vi "Interactive Demo.vi"() -> ()   [LabVIEW 2013, in "dotNETChart XControl.xctl"]
uses:
  dotNETChart XControl.xctl
  typedefs/ChartType.ctl
  typedefs/3DSettings.ctl
  <vilib>/express/express shared/transition.llb/Dynamic To Waveform Array.vi
  <vilib>/express/express signal manip/GetorSetDDTAttributes/Set DDT Attributes/SetT0.vi
  <vilib>/express/express shared/transition.llb/Waveform Array To Dynamic.vi
  <vilib>/express/express signal manip/GetorSetDDTAttributes/Set DDT Attributes/Set DDT Properties.xnode
panel:
  in  "Chart Type 2":i32(ring)=4 caption="Chart Type"
  in  "Series 1 Data Colour":u32(colorbox)=6836 caption="Series Data Colour"
  in  "series name":string="First Series Title" caption="xaxislabel"
  in  "Chart Palette":u16(ring)
  in  "Chart Type":i32(ring)=4
  in  "Chart Wall Gradient Colour":u32(colorbox)=12116479
  in  "Gradient Style":i32(ring)=4
  in  "Chart Wall Border Colour":u32(colorbox)=16777238
  in  "Chart Wall Colour":u32(colorbox)
  in  "chart_wall_trans":u8(slide)=31 caption="Chart Wall Opacity" scale=0.0..255.0
  in  "Legend Style":u16(ring) items=["Column", "Row", "Table"]
  in  "Mouse Zoom":u16(ring)=1 items=["off", "on (2D mode only)"]
  in  "Series 2 Data Colour":u32(colorbox)=12116479 caption="Series Data Colour"
  in  "Skin Style":i32(ring)=1 items=["None", "Emboss", "Raised", "Sunken", "FrameThin1", "FrameThin2", "FrameThin3", "FrameThin4", "FrameThin5", "FrameThin6", "FrameTitle1", "FrameTitle2", "FrameTitle3", "FrameTitle4", "FrameTitle5", "FrameTitle6", "FrameTitle7", "FrameTitle8"]
  in  "yaxislabel":string="Y axis label" caption="xaxislabel"
  in  "xaxislabel":string="X axis label"
  in  "3dmode":bool=TRUE caption="3D Mode"
  in  "Rotation":i32=25
  in  "Wall Width":i32=2
  in  "Perspective":i32=4
  in  "LightStyle":i32(ring)=2 items=["None", "Simplistic", "Realistic"]
  in  "Inclination":i32=21
  in  "Random":bool
  out "dotNETChart XControl":dynamicdata(xcontrol)=[{"t0"=timestamp(3359225754.779551 s since 1904-01-01), "dt"=0.001, "Y"=[-0.21293878372691832, 0.10480719171607178, 0.5198645121842703, 0.4960927860135643, 0.8486500407057044, -0.19156178243419908, -0.3213988951228298, -1.0007275322775073, -1.3720240757016509, -0.2660093892305525, -0.23724681626115568, 0.796814395938406, 0.9778645666014882, 0.7870343306028441, 0.7585739928106939, 0.26409213430431566, -0.8946529385336436, -1.169162891258134, -1.1556662975978256, -0.3690681531689127], "attributes"=variant("NI_ChannelName"=variant(string "First Series Title"), "NI_ExpIsRelativeTime"=variant(bool FALSE), "NI_ExpStartTimeStamp"=variant(timestamp timestamp(3359225754.779551 s since 1904-01-01)), "NI_ExpTimeStamp"=variant(timestamp timestamp(3359225754.779551 s since 1904-01-01)), "NI_ExpXDimension"=variant(string "t"))}, {"t0"=timestamp(3359225754.779551 s since 1904-01-01), "dt"=0.001, "Y"=[-0.22651223041771185, 0.4171889778375242, 0.6017245565566697, 0.9588615672567297, 0.748101089941119, -0.27993796654087566, -0.8863552944000307, -1.0635191133061586, -0.9344284949437466, -0.1710474405944974, 0.3018910917348227, 0.5301156955284767, 1.4475242535659825, 1.1713473149513396, 0.25407740207025176, -0.025061984573477407, -0.48652113815437137, -0.7534989399164532, -1.2184058505207012, -0.10043002227520204], "attributes"=variant("NI_ChannelName"=variant(string "Sine with Uniform Noise"), "NI_ExpIsRelativeTime"=variant(bool FALSE), "NI_ExpStartTimeStamp"=variant(timestamp timestamp(3359225754.779551 s since 1904-01-01)), "NI_ExpTimeStamp"=variant(timestamp timestamp(3359225754.779551 s since 1904-01-01)), "NI_ExpXDimension"=variant(string "t"))}]
  # "Settings"
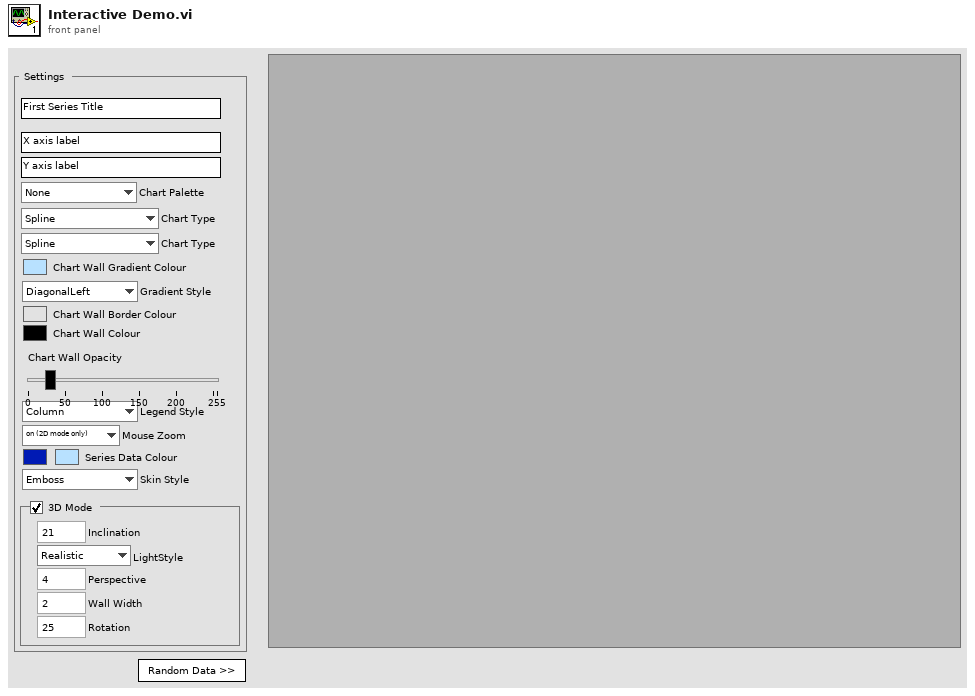
[diagram p1: front panel]
types:
  T1 = typedef "ChartType.ctl" = i32
  T2 = typedef "BackGradientStyle.ctl" = i32
  T3 = typedef "LegendStyle.ctl" = i32
  T4 = typedef "SkinStyle.ctl" = i32
  T5 = typedef "3DSettings.ctl" = cluster{"Inclination":i32, "LightStyle":i32, "Perspective":i32, "WallWidth":i32, "Rotation":i32}
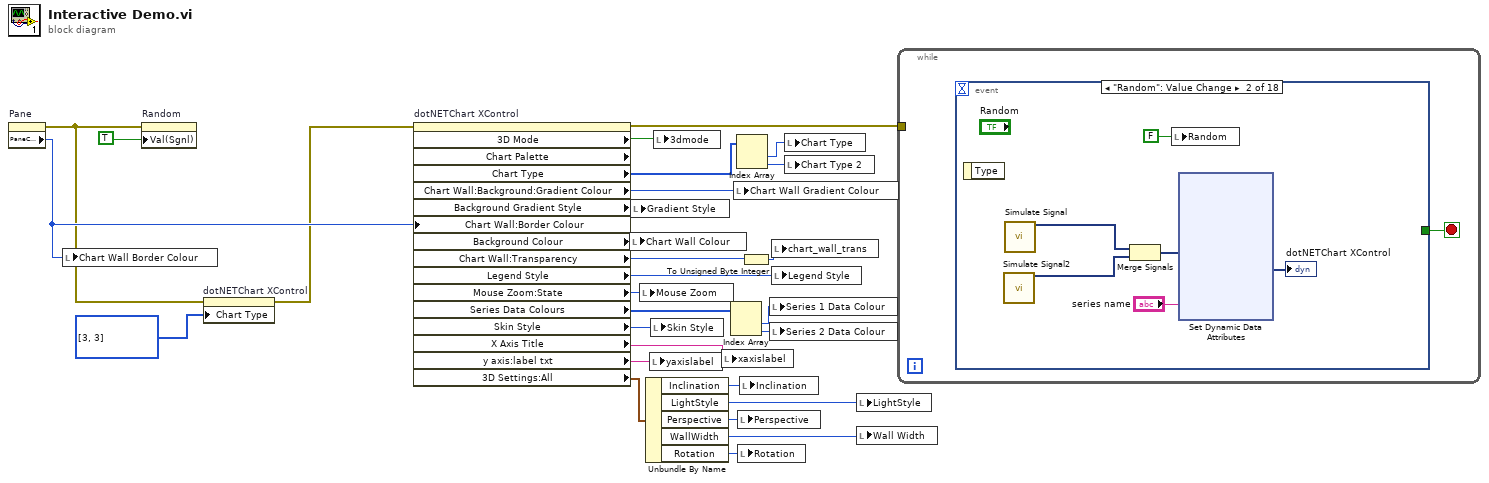
[diagram p0: block diagram]
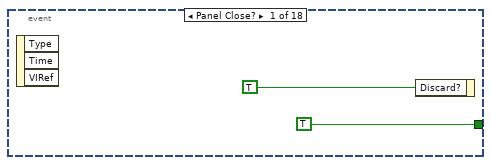
[diagram p2: hidden frame]
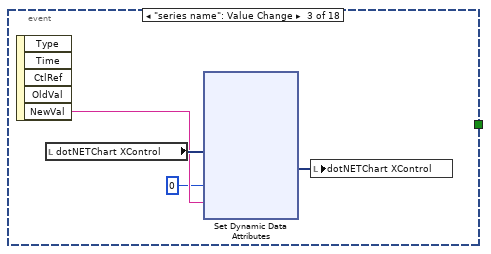
[diagram p3: hidden frame]
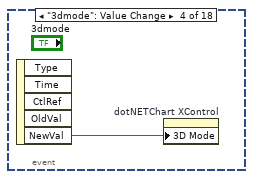
[diagram p4: hidden frame]
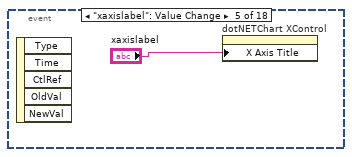
[diagram p5: hidden frame]
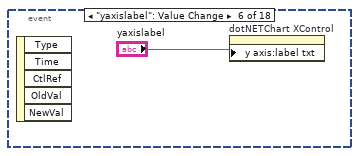
[diagram p6: hidden frame]
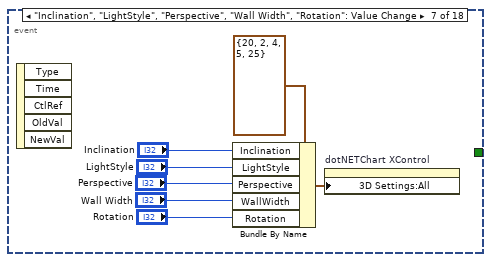
[diagram p7: hidden frame]
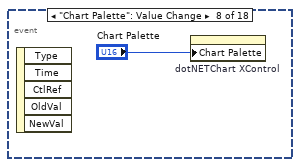
[diagram p8: hidden frame]
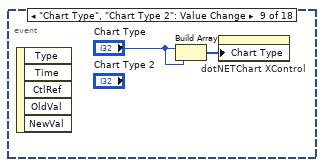
[diagram p9: hidden frame]
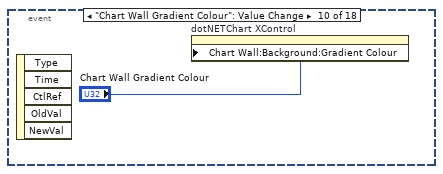
[diagram p10: hidden frame]
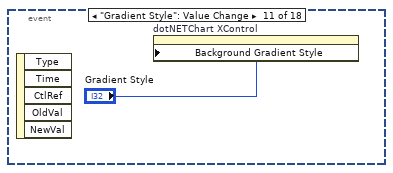
[diagram p11: hidden frame]
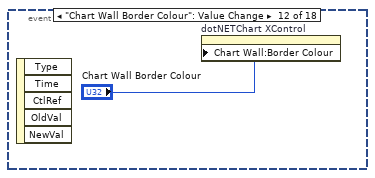
[diagram p12: hidden frame]
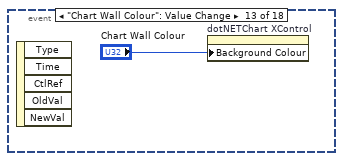
[diagram p13: hidden frame]
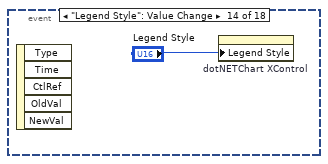
[diagram p14: hidden frame]
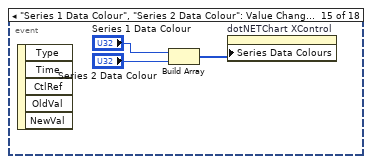
[diagram p15: hidden frame]
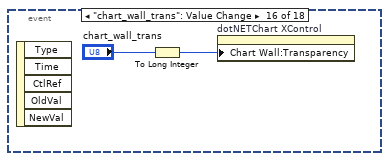
[diagram p16: hidden frame]
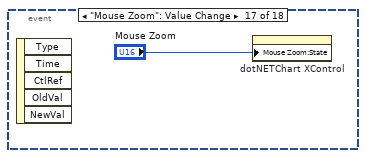
[diagram p17: hidden frame]
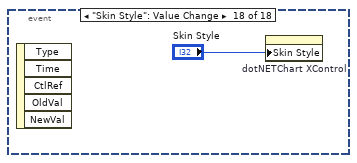
[diagram p18: hidden frame]
diagram:
  w2 = T1[] [3, 3] items=["Point", "FastPoint", "Bubble", "Line", "Spline", "StepLine", "FastLine", "Bar", "StackedBar", "StackedBar100", "Column", "StackedColumn", "StackedColumn100", "Area", "SplineArea", "StackedArea", "StackedArea100", "Pie", "Doughnut", "Stock", "Candlestick", "Range", "SplineRange", "RangeBar", "RangeColumn", "Radar", "Polar", "ErrorBar", "BoxPlot", "Renko", "ThreeLineBreak", "Kagi", "PointAndFigure", "Funnel", "Pyramid"] ("Chart Types")
  n1 = property on="Pane" class="Pane"() -> (error out=w3:errorcluster, "PaneColor"=w7:u32)  [unwired: 2 in, 1 out]
  n2 = local write "Chart Wall Border Colour"(w7) -> ()
  n3 = property on="Random" class="Bool (strict)"(error in=w3, "Val(Sgnl)"=TRUE ("Random")) -> ()  [unwired: 1 in, 2 out]
  n4 = property on="dotNETChart XControl" class="dotNETChart XControl (strict)"(error in=w3, "Chart Type"=w2) -> (error out=w1:errorcluster)  [unwired: 1 in, 1 out]
  n5 = property on="dotNETChart XControl" class="dotNETChart XControl (strict)" props=["3D Mode", "Chart Palette", "Chart Type", "Chart Wall:Background:Gradient Colour", "Background Gradient Style", "Chart Wall:Border Colour", "Background Colour", "Chart Wall:Transparency", "Legend Style", "Mouse Zoom:State", "Series Data Colours", "Skin Style", "X Axis Title", "y axis:label txt", "3D Settings:All"](error in=w1, "Chart Wall:Border Colour"=w7) -> (error out=w28:errorcluster, "3D Mode"=w27:bool, "Chart Type"=w9:T1[], "Chart Wall:Background:Gradient Colour"=w10:u32, "Background Gradient Style"=w11:T2, "Background Colour"=w13:u32, "Chart Wall:Transparency"=w12:i32, "Legend Style"=w15:T3, "Mouse Zoom:State"=w16:enum16{"off", "on (2D mode only)"}, "Series Data Colours"=w17:u32[], "Skin Style"=w18:T4, "X Axis Title"=w20:string, "y axis:label txt"=w19:string, "3D Settings:All"=w26:T5)  [unwired: 1 in, 2 out]
  n6 = local write "Chart Wall Colour"(w13) -> ()
  n7 = local write "Gradient Style"(w11) -> ()
  n8 = local write "Mouse Zoom"(w16) -> ()
  n9 = Unbundle By Name(w26) -> ("Inclination"=w25:i32, "LightStyle"=w24:i32, "Perspective"=w23:i32, "WallWidth"=w22:i32, "Rotation"=w21:i32)
  n10 = local write "yaxislabel"(w19) -> ()
  n11 = local write "Skin Style"(w18) -> ()
  n12 = local write "3dmode"(w27) -> ()
  n13 = local write "xaxislabel"(w20) -> ()
  n14 = Index Array(array=w17) -> (element #1=w5:u32, element #2=w6:u32)  [unwired: 2 in]
  n15 = local write "Chart Wall Gradient Colour"(w10) -> ()
  n16 = Index Array(array=w9) -> (element #1=w8:T1, element #2=w4:T1)  [unwired: 2 in]
  n17 = local write "Perspective"(w23) -> ()
  n18 = local write "Rotation"(w21) -> ()
  n19 = local write "Inclination"(w25) -> ()
  n20 = To Unsigned Byte Integer(number=w12) -> (unsigned 8bit integer=w14:u8)
  n21 = local write "Series 1 Data Colour"(w5) -> ()
  n22 = local write "Series 2 Data Colour"(w6) -> ()
  n23 = local write "chart_wall_trans"(w14) -> ()
  n24 = local write "Legend Style"(w15) -> ()
  n25 = local write "Chart Type"(w8) -> ()
  n26 = local write "Chart Type 2"(w4) -> ()
  n27 = local write "LightStyle"(w24) -> ()
  n28 = local write "Wall Width"(w22) -> ()
  n29 = while {
    tunnel: w28 -> [_]
    stop <- w30 stop-if-true
    n30 = event shown="[1] \"Random\": Value Change" {
      selector: _ -> [_ _ _ _ _ _ _ _ _ _ _ _ _ _ _ _ _ _]
      dyn-events: _ -> [_ _ _ _ _ _ _ _ _ _ _ _ _ _ _ _ _ _]
      timeout: _ -> [_ _ _ _ _ _ _ _ _ _ _ _ _ _ _ _ _ _]
      tunnel: [TRUE _ _ _ _ _ _ _ _ _ _ _ _ _ _ _ _ _] -> w30
      event Panel Close? {
        n31 = event-data() -> ()  [unwired: 1 in, 3 out]
        n32 = event-data("Discard?"=TRUE) -> ()  [unwired: 1 in, 1 out]
      }
      event "Random": Value Change {
        n33 = event-data() -> ()  [unwired: 1 in, 1 out]
        n34 = call "Simulate Signal2"() -> ("Sine with Uniform Noise"=w33:dynamicdata)  [unwired: 14 in, 1 out]
        n35 = call "Simulate Signal"() -> ("Sine with Uniform Noise"=w38:dynamicdata)  [unwired: 14 in, 1 out]
        n36 = Merge Signals(w38, w33) -> (w34:dynamicdata)
        n37 = local write "Random"(FALSE ("Random")) -> ()
        n38 = xnode "Set Dynamic Data Attributes"("Signals In"=w34, "Signal Name"="series name") -> ("Signals Out"=→"dotNETChart XControl":dynamicdata)  [unwired: 2 in, 1 out]
      }
      event "series name": Value Change {
        n39 = event-data() -> ("NewVal"=w54:string)  [unwired: 1 in, 4 out]
        n40 = local read "dotNETChart XControl"() -> (w55:dynamicdata)
        n41 = xnode "Set Dynamic Data Attributes"("Signals In"=w55, "Signal Index"=0, "Signal Name"=w54) -> ("Signals Out"=w56:dynamicdata)  [unwired: 1 in, 1 out]
        n42 = local write "dotNETChart XControl"(w56) -> ()
      }
      event "3dmode": Value Change {
        n43 = event-data() -> ("NewVal"=w70:bool)  [unwired: 1 in, 4 out]
        n44 = property on="dotNETChart XControl" class="dotNETChart XControl (strict)"("3D Mode"=w70) -> ()  [unwired: 2 in, 2 out]
      }
      event "xaxislabel": Value Change {
        n45 = event-data() -> ()  [unwired: 1 in, 5 out]
        n46 = property on="dotNETChart XControl" class="dotNETChart XControl (strict)"("X Axis Title"="xaxislabel") -> ()  [unwired: 2 in, 2 out]
      }
      event "yaxislabel": Value Change {
        n47 = event-data() -> ()  [unwired: 1 in, 5 out]
        n48 = property on="dotNETChart XControl" class="dotNETChart XControl (strict)"("y axis:label txt"="yaxislabel") -> ()  [unwired: 2 in, 2 out]
      }
      event "Inclination", "LightStyle", "Perspective", "Wall Width", "Rotation": Value Change {
        n49 = event-data() -> ()  [unwired: 1 in, 5 out]
        n50 = Bundle By Name(cluster=T5 {"Inclination"=20, "LightStyle"=2, "Perspective"=4, "WallWidth"=5, "Rotation"=25} ("3D Settings:All Elements"), "Inclination"="Inclination", "LightStyle"="LightStyle", "Perspective"="Perspective", "WallWidth"="Wall Width", "Rotation"="Rotation") -> (w78:T5)
        n51 = property on="dotNETChart XControl" class="dotNETChart XControl (strict)"("3D Settings:All"=w78) -> ()  [unwired: 2 in, 2 out]
      }
      event "Chart Palette": Value Change {
        n52 = event-data() -> ()  [unwired: 1 in, 5 out]
        n53 = property on="dotNETChart XControl" class="dotNETChart XControl (strict)"("Chart Palette"="Chart Palette") -> ()  [unwired: 2 in, 2 out]
      }
      event "Chart Type", "Chart Type 2": Value Change {
        n54 = event-data() -> ()  [unwired: 1 in, 5 out]
        n55 = Build Array("Chart Type", "Chart Type") -> (w82:i32[])
        n56 = property on="dotNETChart XControl" class="dotNETChart XControl (strict)"("Chart Type"=w82) -> ()  [unwired: 2 in, 2 out]
      }
      event "Chart Wall Gradient Colour": Value Change {
        n57 = event-data() -> ()  [unwired: 1 in, 5 out]
        n58 = property on="dotNETChart XControl" class="dotNETChart XControl (strict)"("Chart Wall:Background:Gradient Colour"="Chart Wall Gradient Colour") -> ()  [unwired: 2 in, 2 out]
      }
      event "Gradient Style": Value Change {
        n59 = event-data() -> ()  [unwired: 1 in, 5 out]
        n60 = property on="dotNETChart XControl" class="dotNETChart XControl (strict)"("Background Gradient Style"="Gradient Style") -> ()  [unwired: 2 in, 2 out]
      }
      event "Chart Wall Border Colour": Value Change {
        n61 = event-data() -> ()  [unwired: 1 in, 5 out]
        n62 = property on="dotNETChart XControl" class="dotNETChart XControl (strict)"("Chart Wall:Border Colour"="Chart Wall Border Colour") -> ()  [unwired: 2 in, 2 out]
      }
      event "Chart Wall Colour": Value Change {
        n63 = event-data() -> ()  [unwired: 1 in, 5 out]
        n64 = property on="dotNETChart XControl" class="dotNETChart XControl (strict)"("Background Colour"="Chart Wall Colour") -> ()  [unwired: 2 in, 2 out]
      }
      event "Legend Style": Value Change {
        n65 = event-data() -> ()  [unwired: 1 in, 5 out]
        n66 = property on="dotNETChart XControl" class="dotNETChart XControl (strict)"("Legend Style"="Legend Style") -> ()  [unwired: 2 in, 2 out]
      }
      event "Series 1 Data Colour", "Series 2 Data Colour": Value Change {
        n67 = event-data() -> ()  [unwired: 1 in, 5 out]
        n68 = Build Array("Series 1 Data Colour", "Series 2 Data Colour") -> (w90:u32[])
        n69 = property on="dotNETChart XControl" class="dotNETChart XControl (strict)"("Series Data Colours"=w90) -> ()  [unwired: 2 in, 2 out]
      }
      event "chart_wall_trans": Value Change {
        n70 = event-data() -> ()  [unwired: 1 in, 5 out]
        n71 = To Long Integer(number="chart_wall_trans") -> (32bit integer=w91:i32)
        n72 = property on="dotNETChart XControl" class="dotNETChart XControl (strict)"("Chart Wall:Transparency"=w91) -> ()  [unwired: 2 in, 2 out]
      }
      event "Mouse Zoom": Value Change {
        n73 = event-data() -> ()  [unwired: 1 in, 5 out]
        n74 = property on="dotNETChart XControl" class="dotNETChart XControl (strict)"("Mouse Zoom:State"="Mouse Zoom") -> ()  [unwired: 2 in, 2 out]
      }
      event "Skin Style": Value Change {
        n75 = event-data() -> ()  [unwired: 1 in, 5 out]
        n76 = property on="dotNETChart XControl" class="dotNETChart XControl (strict)"("Skin Style"="Skin Style") -> ()  [unwired: 2 in, 2 out]
      }
    }
  }
